vi "ForLoops_IndexingExample_NoteDisplayTiming.vi"() -> ()   [LabVIEW 2019]
panel:
  out "Array 2":i32[](array[numeric])
  out "Numeric":i32
  out "Array":i32[](array[numeric])
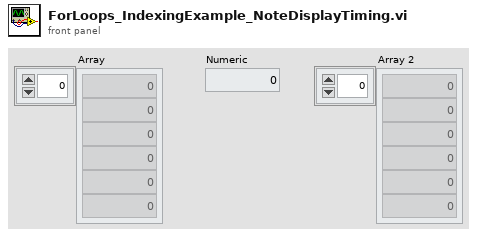
[diagram p1: front panel]
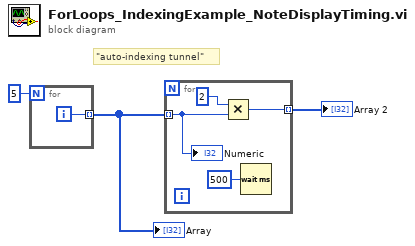
[diagram p0: block diagram]
diagram:
  # "\"auto-indexing tunnel\""
  n1 = for {
    N: 5 -> [_]
    tunnel: [w4] -> w2 mode=indexing
    i -> [w4]
  }
  "Array" <- w2
  n2 = for {
    tunnel: w2 -> [w7] mode=indexing
    tunnel: [w5] -> w1 mode=indexing
    n3 = Multiply(x=2, y=w7) -> (x*y=w5:i32)
    n4 = Wait (ms)(milliseconds to wait=u32 500) -> ()  [unwired: 1 out]
    "Numeric" <- w7
  }
  "Array 2" <- w1
